vi "Lab2.vi"() -> ()   [LabVIEW 2010]
uses:
  <vilib>/Utility/file.llb/Write To Spreadsheet File (DBL).vi
  <vilib>/Analysis/NI_AALBase.lvlib
panel:
  in  "Save?":bool
  in  "intervals":i32=10
  out "XY Graph":T1(graph)
  out "Waveform Graph":dbl[](graph)
  in  "Desired Expected random number":dbl
  in  "Number of random numbers":dbl
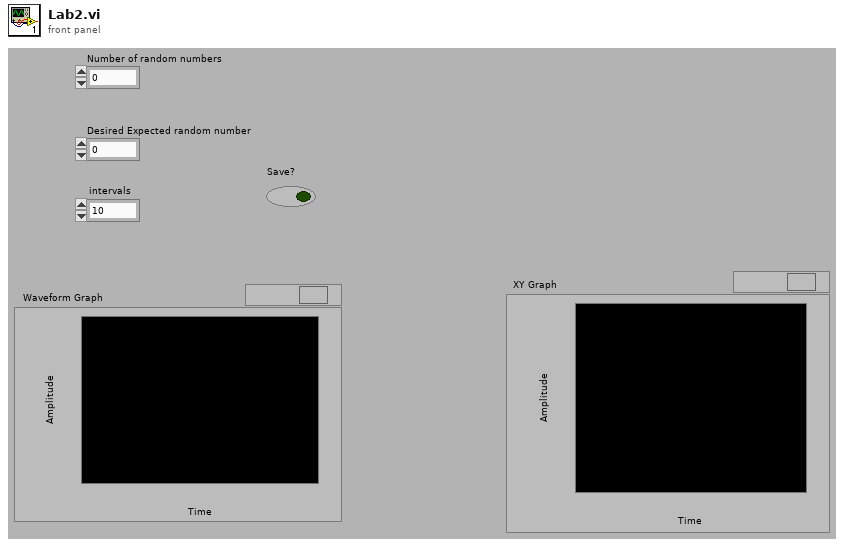
[diagram p1: front panel]
types:
  T1 = cluster{"X Values":dbl[], "Histogram: h(x)":i32[]}
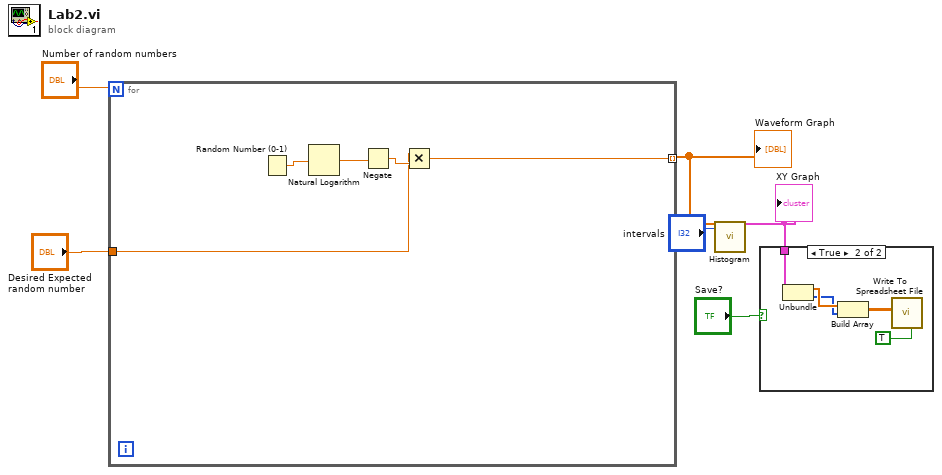
[diagram p0: block diagram]
diagram:
  n1 = for {
    N: "Number of random numbers" -> [_]
    tunnel: "Desired Expected random number" -> [w7]
    tunnel: [w8] -> w3 mode=indexing
    n2 = Random Number (0-1)() -> (number: 0 to 1=w9:dbl)
    n3 = Natural Logarithm(1:w9) -> (0:w10:dbl)
    n4 = Negate(x=w10) -> (-x=w11:dbl)
    n5 = Multiply(x=w7, y=w11) -> (x*y=w8:dbl)
  }
  "Waveform Graph" <- w3
  n6 = call <vilib>:"Histogram.vi"("intervals"="intervals", "X"=w3) -> ("Histogram Graph"=w2:T1)  [unwired: 6 in, 3 out]
  "XY Graph" <- w2
  n7 = case shown="True" "Save?" {
    tunnel: w2 -> [_ w15]
    frame False {
    }
    frame True {
      n8 = Unbundle(w15) -> ("X Values"=w14:dbl[], "Histogram: h(x)"=w13:i32[])
      n9 = Build Array(w14, w13) -> (w12:dbl[][])
      n10 = call-poly <vilib>:"Write To Spreadsheet File.vi"("transpose? (no:F)"=TRUE, "2D data"=w12) -> ()  [unwired: 6 in, 1 out]
    }
  }
